vi "Get Cursor Position.vi"() -> (2 "CursorX":i32, 3 "CursorY":i32)   [LabVIEW 2015]
uses:
  user32.dll
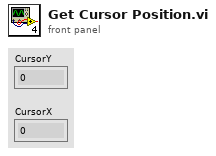
[diagram p1: front panel]
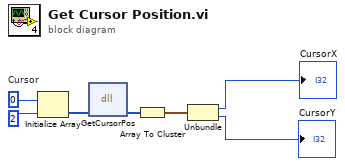
[diagram p0: block diagram]
diagram:
  w5 = 0  # Cursor
  n1 = Initialize Array(w5, 2) -> (w2:i32[])
  n2 = dll-call lib="user32.dll" fn="GetCursorPos"("POINT"=w2) -> ("POINT"=w3:i32[])  [unwired: 4 in, 2 out]
  n3 = Array To Cluster(array=w3) -> (cluster=w1:cluster{"POINT[0]":i32, "POINT[1]":i32})
  n4 = Unbundle(w1) -> ("POINT[0]"=→"CursorX":i32, "POINT[1]"=→"CursorY":i32)
